vi "Get DataRate.vi"(8 "error in (no error)":errorcluster, 11 "TLCamera reference in":refnum<k24>) -> (0 "error out":errorcluster, 2 "DataRate":T1, 3 "TLCamera reference out":refnum<k24>)   [LabVIEW 2015]
uses:
  C:/code/Host/Installer/Scientific Camera Interfaces/LabVIEW/32_bit/Library_X86/Thorlabs.TSI.TLCameraInterfaces.dll
  32_bit/Library_X86/Thorlabs.TSI.TLCameraInterfaces.dll
  Controls/Data Rate.ctl
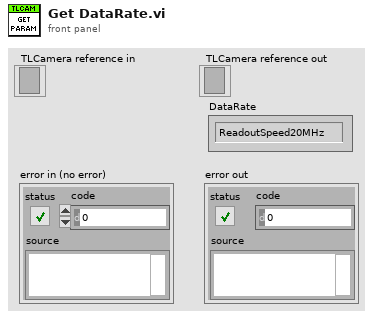
[diagram p1: front panel]
types:
  T1 = typedef "Data Rate.ctl" = enum32{"ReadoutSpeed20MHz", "ReadoutSpeed40MHz", "FPS30", "FPS50"}
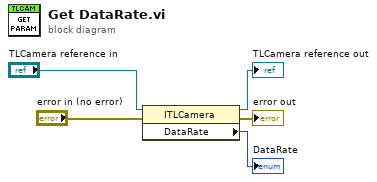
[diagram p0: block diagram]
diagram:
  n1 = property class="ITLCamera"(reference="TLCamera reference in", error in="error in (no error)") -> (reference out=→"TLCamera reference out":refnum<k24>, error out=→"error out":errorcluster, "DataRate"=→"DataRate":i32)
